vi "Jump Back.vi"(8 "error in":errorcluster, 10 "VI Name":string, 11 "Data Cluster":T1) -> (0 "error out":errorcluster, 3 "Module Data":T1)   [LabVIEW 2020, in "Peek Window.lvlib"]
uses:
  Peek Window.lvlib
  MHL Data Cluster.ctl
  Open Diagram Argument--cluster.ctl
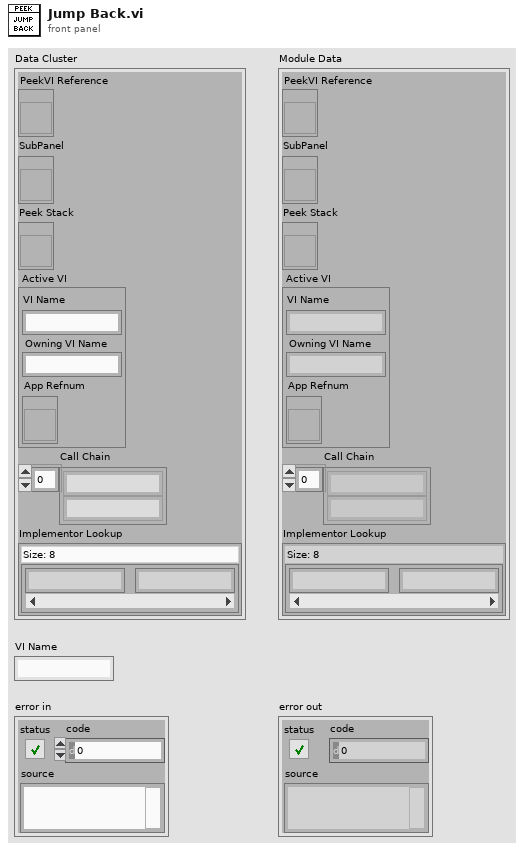
[diagram p1: front panel]
types:
  T1 = typedef "Peek Window.lvlib/MHL Data Cluster.ctl" = cluster{"PeekVI Reference":refnum<vi>, "SubPanel":refnum<vi>, "Peek Stack":refnum<vi>, "Active VI":T2, "Call Chain":string[], "Implementor Lookup":map{string, string}}
  T2 = typedef "Peek Window.lvlib/Open Diagram Argument--cluster.ctl" = cluster{"VI Name":string, "Owning VI Name":string, "App Refnum":refnum<vi>}
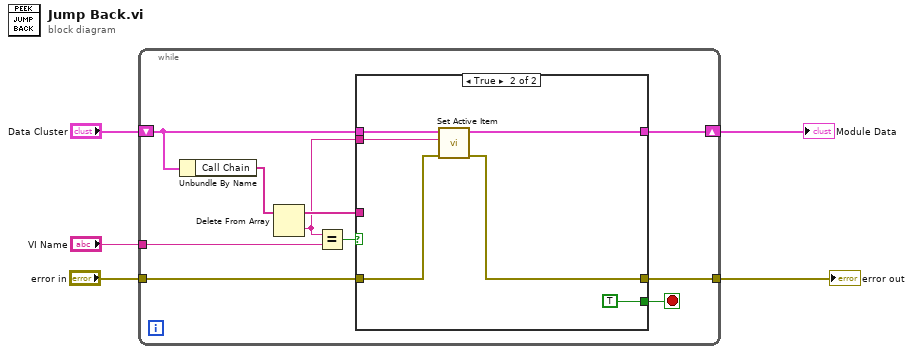
[diagram p0: block diagram]
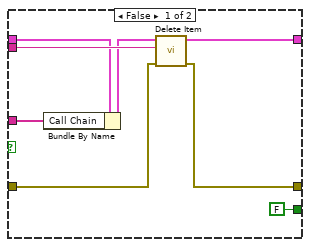
[diagram p2: hidden frame]
diagram:
  n1 = while {
    tunnel: "error in" -> [w10]
    tunnel: [w11] -> w2
    tunnel: "VI Name" -> [w15]
    shift-right: [w13] -> w4
    shift-left: "Data Cluster" -> [w12]
    stop <- w8 stop-if-true
    n2 = Unbundle By Name(w12) -> ("Call Chain"=w9:string[])
    n3 = Delete From Array(array=w9) -> (deleted portion=w6:string, array with subset deleted=w7:string[])  [unwired: 2 in]
    n4 = Equal?(x=w6, y=w15) -> (x = y?=w14:bool)
    n5 = case shown="True" w14 {
      tunnel: [w18 w28] -> w13
      tunnel: w12 -> [w16 w27]
      tunnel: [w22 w25] -> w11
      tunnel: w10 -> [w23 w24]
      tunnel: w7 -> [w21 _]
      tunnel: [FALSE TRUE] -> w8
      tunnel: w6 -> [w19 w26]
      frame False {
        n6 = Bundle By Name(cluster=w16, "Call Chain"=w21) -> (w17:T1)
        n7 = call "Delete Item.vi"("error in (no error)"=w23, "Removed VI"=w19, "Data Cluster"=w17) -> ("error out"=w22:errorcluster, "Module Data"=w18:T1)  [unwired: 7 in]
      }
      frame True {
        n8 = call "Set Active Item.vi"("error in (no error)"=w24, "Active VI"=w26, "Data Cluster"=w27) -> ("error out"=w25:errorcluster, "Module Data"=w28:T1)  [unwired: 7 in]
      }
    }
  }
  "Module Data" <- w4
  "error out" <- w2
